vi "GrapRealTimeData.vi"(11 "Code":string="sz002195") -> (3 "Grab Data":string)   [LabVIEW 2013]
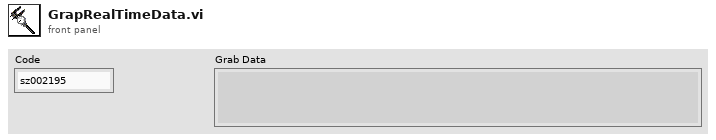
[diagram p1: front panel]
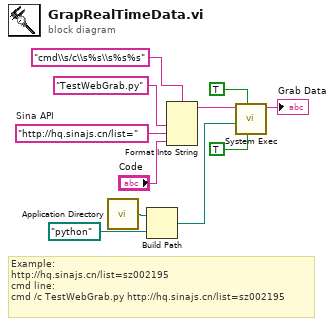
[diagram p0: block diagram]
diagram:
  w3 = "http://hq.sinajs.cn/list="  # Sina API
  # "Example:\nhttp://hq.sinajs.cn/list=sz002195\ncmd line:\ncmd /c TestWebGrab.py http://hq.sinajs.cn/list=sz002195"
  n1 = call <vilib>:"Application Directory.vi"() -> ("Application Directory"=w7:path)
  n2 = Build Path(base path=w7, name or relative path=path "python" ("working directory")) -> (appended path=w5:path)
  n3 = Format Into String(format string="cmd\\s/c\\s%s\\s%s%s", "TestWebGrab.py" ("input 1"), w3, "Code") -> (resulting string=w8:string)  [unwired: 2 in, 1 out]
  n4 = call <vilib>:"System Exec.vi"("run minimized? (F)"=TRUE, "wait until completion? (T)"=TRUE, "working directory"=w5, "command line"=w8) -> ("standard output"=→"Grab Data":string)  [unwired: 4 in, 3 out]
